vi "Untitled 1 (SubVI).vi"(8 "error in (no error)":errorcluster, 11 "String in":string) -> (0 "error out":errorcluster, 3 "TileNumber":u16)   [LabVIEW 2019, in "RT_Game.lvlib" / "SnakeGame.lvclass"]
uses:
  SnakeGame.lvclass
  Game/Game.lvclass
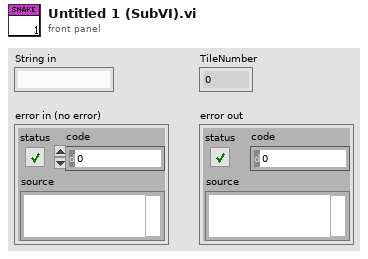
[diagram p1: front panel]
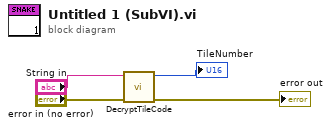
[diagram p0: block diagram]
diagram:
  n1 = call "DecryptTileCode.vi"("error in (no error)"="error in (no error)", "TileCode"="String in") -> ("error out"=→"error out":errorcluster, "TileCode"=→"TileNumber":u16)  [unwired: 6 in, 2 out]
